vi "Start Utilization HTTP.vi"(8 "error in (no error)":errorcluster, 10 "configuration":refnum<class "NI Skyline Configuration HTTP.lvclass">, 11 "asset":T1) -> (0 "error out":errorcluster, 2 "utilizationIdentifier":string, 3 "JSON string":string)   [LabVIEW 2023, in "Logger.lvclass"]
uses:
  Logger.lvclass
  <vilib>/Skyline/Configuration/Configuration HTTP_class/NI Skyline Configuration HTTP.lvclass
  <vilib>/Skyline/Configuration/Configuration HTTP_class/NI Skyline Configuration HTTP.lvclass/NI Skyline Configuration HTTP.ctl
  <vilib>/Skyline/Configuration/Configuration HTTP_class/Read Server URL.vi
  <vilib>/httpClient/POSTBuffer.vi
  <vilib>/httpClient/LabVIEWHTTPClient.lvlib
  <vilib>/Skyline/Utilities/NI Skyline Utilities.lvlib
panel:
  out "URL":string
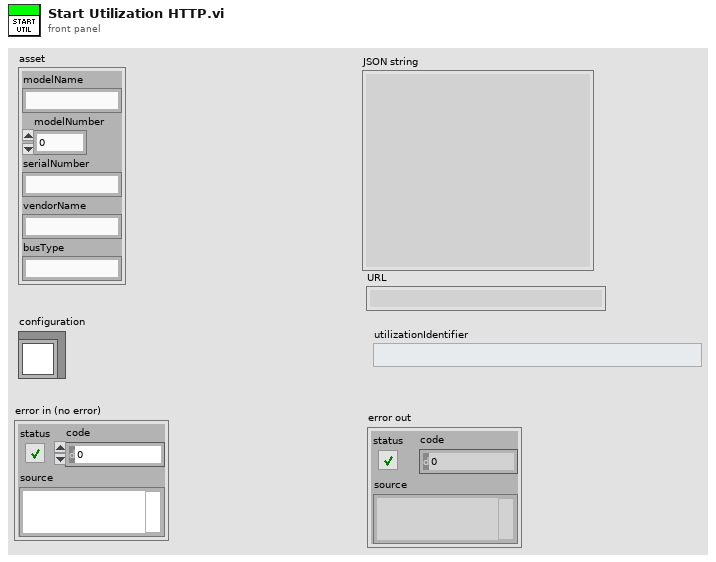
[diagram p1: front panel]
types:
  T1 = cluster{"modelName":string, "modelNumber":i32, "serialNumber":string, "vendorName":string, "busType":string}
  T2 = cluster{"utilizationIdentifier":string, "minionId":string, "assetIdentifications":cluster{"modelName":string, "modelNumber":i32, "serialNumber":string, "vendorName":string, "busType":string}[], "utilizationCategory":string, "taskName":string, "userName":string, "utilizationTimestamp":string}
  T3 = cluster{"modelName":string, "modelNumber":i32, "serialNumber":string, "vendorName":string, "busType":string}[]
  T4 = typedef "LabVIEWHTTPClient.lvlib/ClientHandle.ctl" = refnum<k1>
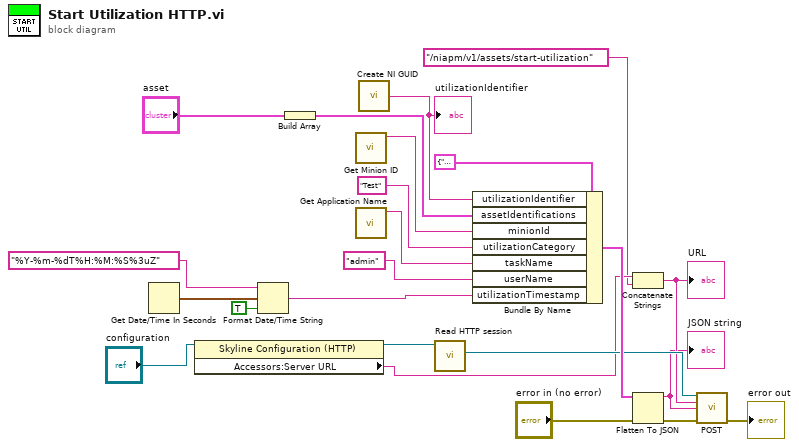
[diagram p0: block diagram]
diagram:
  n1 = Get Date/Time In Seconds() -> (seconds since 1Jan1904=w16:timestamp)
  n2 = property class="Skyline Configuration (HTTP)"(reference="configuration") -> (reference out=w9:refnum<class "NI Skyline Configuration HTTP.lvclass">, "Accessors:Server URL"=w7:string)  [unwired: 1 in, 1 out]
  n3 = Format Date/Time String(time format string (%c)="%Y-%m-%dT%H:%M:%S%3uZ", seconds (now)=w16, UTC format=TRUE) -> (date/time string=w19:string)
  n4 = Build Array("asset") -> (w14:T3)
  n5 = call <vilib>:"Get Minion ID.vi"() -> ("minion id"=w15:string)  [unwired: 11 in]
  n6 = call "Get Application Name.vi"() -> ("Application"=w20:string)  [unwired: 11 in]
  n7 = call <vilib>:"Create NI GUID.vi"() -> ("NI GUID"=w1:string)
  "utilizationIdentifier" <- w1
  n8 = call <vilib>:"Read HTTP session.vi"("HTTP configuration in"=w9) -> ("http session"=w8:T4)  [unwired: 8 in, 2 out]
  n9 = Bundle By Name(cluster=T2 {"utilizationIdentifier"="", "minionId"="", "assetIdentifications"=[], "utilizationCategory"="", "taskName"="", "userName"="", "utilizationTimestamp"=""}, "utilizationIdentifier"=w1, "assetIdentifications"=w14, "minionId"=w15, "utilizationCategory"="Test", "taskName"=w20, "userName"="admin", "utilizationTimestamp"=w19) -> (w13:T2)
  n10 = Concatenate Strings(w7, "/niapm/v1/assets/start-utilization") -> (w5:string)
  "URL" <- w5
  n11 = Flatten To JSON(anything=w13, error in (no error)="error in (no error)") -> (JSON string=w4:string, 11:w3:errorcluster)  [unwired: 1 in]
  "JSON string" <- w4
  n12 = call-poly <vilib>:"POST.vi"("client handle"=w8, "url"=w5, "buffer"=w4, "error in (no error)"=w3) -> ("error out"=→"error out":errorcluster)  [unwired: 8 in, 3 out]
